vi "Twin_Simulator.vi"(6 "L2":dbl=130.0, 7 "L1":dbl=100.0, 8 "origin":cluster{"X":dbl, "Y":dbl}={"X"=200.0, "Y"=250.0}, 9 "a":dbl=20.0, 10 "beta 2":dbl(slide)=137.76536312849163 scale=-180.0..180.0, 11 "beta 1":dbl(slide)=43.24022346368716 scale=-180.0..180.0) -> (1 "3D Picture":refnum<vi>(3d-picture), 3 "Canvas":picture)   [LabVIEW 2022 SP3]
panel:
  out "A":dbl=0.009007395105217966
  out "B":dbl=1.2833295473119142
  out "L":dbl=1.2833611573405141
  out "gamma1":dbl=49.705808953024054
  out "gamma2":dbl=50.510495500567416
  out "sigma":dbl=79.87499415983615
  out "theta":dbl=0.4023432737716799
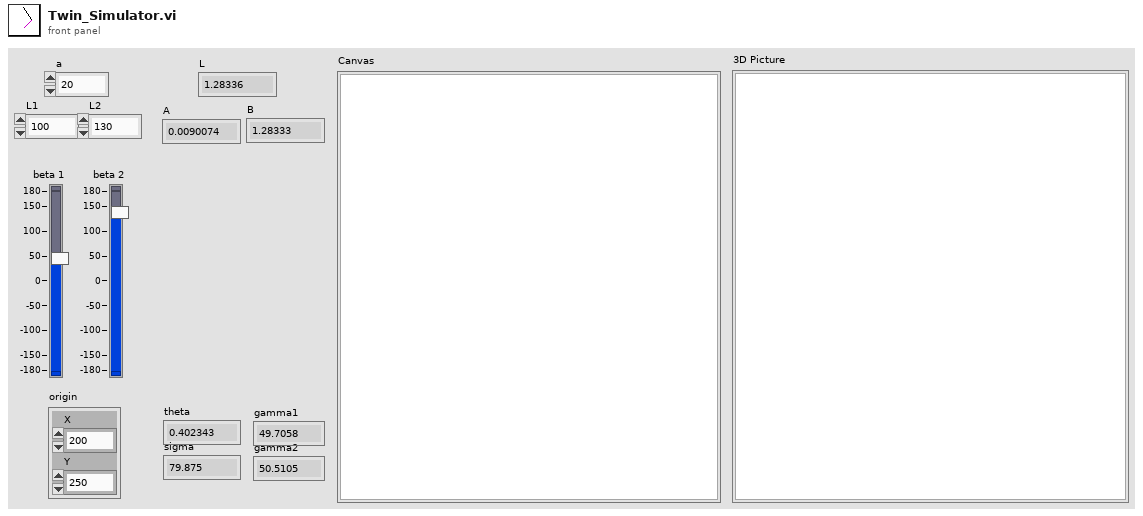
[diagram p1: front panel]
types:
  T1 = cluster{"Color":u32, "Length":dbl, "Base position":cluster{"X":dbl, "Y":dbl}, "Joint Angle":dbl}
  T2 = cluster{"Color":u32, "Length":dbl, "Base position":cluster{"X":dbl, "Y":dbl}, "Joint Angle":dbl}[]
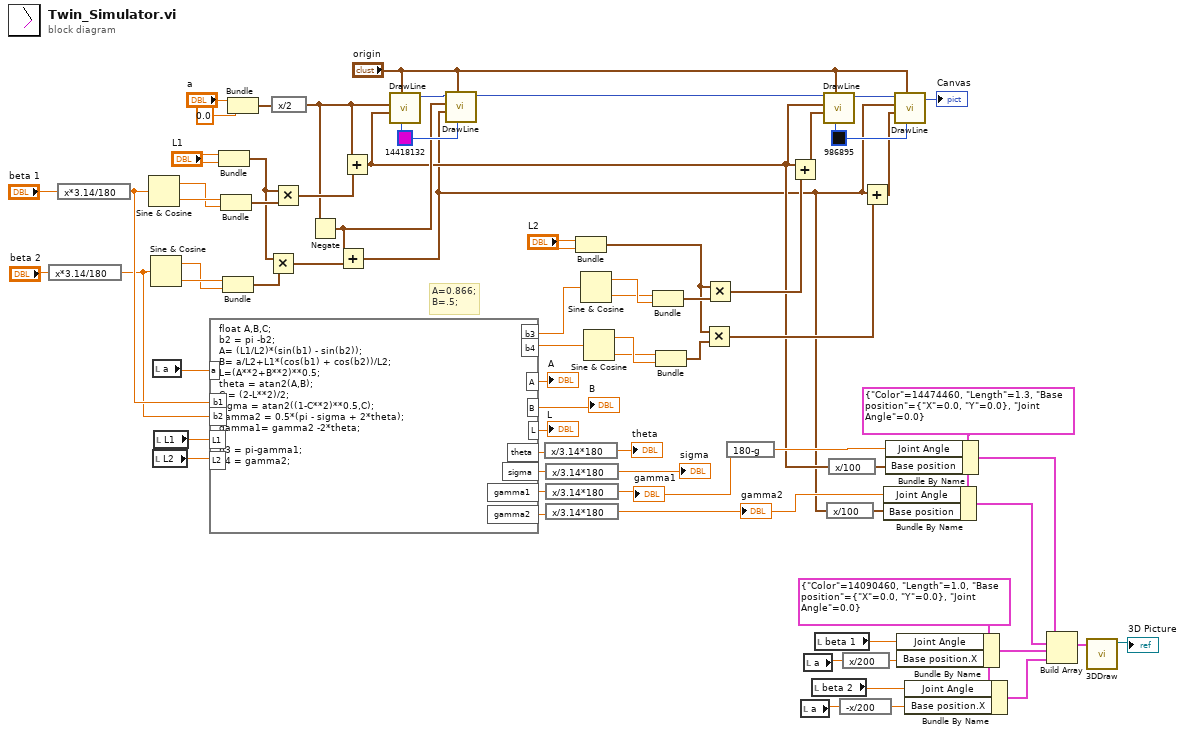
[diagram p0: block diagram]
diagram:
  w10 = T1 {"Color"=14474460, "Length"=1.3, "Base position"={"X"=0.0, "Y"=0.0}, "Joint Angle"=0.0} ("Arm")
  w14 = T1 {"Color"=14090460, "Length"=1.0, "Base position"={"X"=0.0, "Y"=0.0}, "Joint Angle"=0.0} ("Arm")
  w28 = u32 986895 ("color(black)")
  w30 = u32 14418132 ("color(black)")
  # "A=0.866;\nB=.5;"
  n1 = expression code="x*3.14/180"("beta 2") -> (w54:dbl)
  n2 = expression code="x*3.14/180"("beta 1") -> (w55:dbl)
  n3 = Sine & Cosine(0:w55) -> (1:w66:dbl, 2:w67:dbl)
  n4 = Sine & Cosine(0:w54) -> (1:w61:dbl, 2:w62:dbl)
  n5 = local read "a"() -> (w58:dbl)
  n6 = local read "L2"() -> (w56:dbl)
  n7 = local read "L1"() -> (w57:dbl)
  n8 = formula code="float A,B,C;\nb2 = pi -b2;\nA= (L1/L2)*(sin(b1) - sin(b2));\nB= a/L2+L1*(cos(b1) + cos(b2))/L2;\nL=(A**2+B**2)**0.5;\ntheta = atan2(A,B);\nC = (2-L**2)/2;\nsigma = atan2((1-C**2)**0.5,C);\ngamma2 = 0.5*(pi - sigma + 2*theta);\ngamma1= gamma2 -2*theta;\n\nb3 = pi-gamma1;\nb4 = gamma2;"("b1"=w55, "b2"=w54, "L1"=w57, "L2"=w56, "a"=w58) -> ("A"=→"A":dbl, "B"=→"B":dbl, "L"=→"L":dbl, "theta"=w53:dbl, "sigma"=w50:dbl, "gamma1"=w49:dbl, "gamma2"=w48:dbl, "b3"=w40:dbl, "b4"=w39:dbl)
  n9 = Bundle("L1"="L1", "L1"="L1") -> (w59:cluster{"L1":dbl, "L1":dbl})  [unwired: 1 in]
  n10 = Bundle(w67, w66) -> (w65:cluster{dbl, dbl})  [unwired: 1 in]
  n11 = Bundle(w62, w61) -> (w63:cluster{dbl, dbl})  [unwired: 1 in]
  n12 = Bundle("a"="a", 0.0) -> (w69:cluster{"a":dbl, dbl})  [unwired: 1 in]
  n13 = Multiply(x=w59, y=w63) -> (x*y=w37:cluster{dbl, dbl})
  n14 = expression code="x/2"(w69) -> (w32:cluster{"a":dbl, dbl})
  n15 = Multiply(x=w59, y=w65) -> (x*y=w64:cluster{dbl, dbl})
  n16 = Negate(x=w32) -> (-x=w29:cluster{"a":dbl, dbl})
  n17 = Add(x=w29, y=w37) -> (x+y=w1:cluster{dbl, dbl})
  n18 = Add(x=w32, y=w64) -> (x+y=w2:cluster{dbl, dbl})
  n19 = call "DrawLine.vi"("color(black)"=w30, "offset"="origin", "move"=w2, "start"=w32) -> ("picture out"=w31:picture)  [unwired: 7 in]
  n20 = call "DrawLine.vi"("color(black)"=w30, "offset"="origin", "move"=w1, "start"=w29, "picture in"=w31) -> ("picture out"=w26:picture)  [unwired: 6 in]
  n21 = expression code="x/3.14*180"(w53) -> (→"theta":dbl)
  n22 = expression code="x/3.14*180"(w50) -> (→"sigma":dbl)
  n23 = expression code="x/3.14*180"(w49) -> (w4:dbl)
  "gamma1" <- w4
  n24 = expression code="x/3.14*180"(w48) -> (w9:dbl)
  "gamma2" <- w9
  n25 = Bundle("L2"="L2", "L2"="L2") -> (w41:cluster{"L2":dbl, "L2":dbl})  [unwired: 1 in]
  n26 = Sine & Cosine(0:w40) -> (1:w43:dbl, 2:w42:dbl)
  n27 = Sine & Cosine(0:w39) -> (1:w47:dbl, 2:w46:dbl)
  n28 = Bundle(w42, w43) -> (w44:cluster{dbl, dbl})  [unwired: 1 in]
  n29 = Bundle(w46, w47) -> (w45:cluster{dbl, dbl})  [unwired: 1 in]
  n30 = Multiply(x=w41, y=w45) -> (x*y=w36:cluster{dbl, dbl})
  n31 = Multiply(x=w41, y=w44) -> (x*y=w38:cluster{dbl, dbl})
  n32 = expression code="180-g"(w4) -> (w3:dbl)
  n33 = Add(x=w2, y=w38) -> (x+y=w24:cluster{dbl, dbl})
  n34 = local read "a"() -> (w16:dbl)
  n35 = local read "a"() -> (w19:dbl)
  n36 = local read "beta 2"() -> (w15:dbl)
  n37 = local read "beta 1"() -> (w20:dbl)
  n38 = call "DrawLine.vi"("color(black)"=w28, "offset"="origin", "move"=w24, "start"=w2, "picture in"=w26) -> ("picture out"=w27:picture)  [unwired: 6 in]
  n39 = expression code="x/100"(w1) -> (w6:cluster{dbl, dbl})
  n40 = expression code="x/100"(w2) -> (w5:cluster{dbl, dbl})
  n41 = expression code="-x/200"(w16) -> (w17:dbl)
  n42 = expression code="x/200"(w19) -> (w18:dbl)
  n43 = Add(x=w1, y=w36) -> (x+y=w23:cluster{dbl, dbl})
  n44 = Bundle By Name(cluster=w10, "Joint Angle"=w9, "Base position"=w6) -> (w7:T1)
  n45 = Bundle By Name(cluster=w10, "Joint Angle"=w3, "Base position"=w5) -> (w8:T1)
  n46 = call "DrawLine.vi"("color(black)"=w28, "offset"="origin", "move"=w23, "start"=w1, "picture in"=w27) -> ("picture out"=→"Canvas":picture)  [unwired: 6 in]
  n47 = Bundle By Name(cluster=w14, "Joint Angle"=w20, "Base position.X"=w18) -> (w13:T1)
  n48 = Bundle By Name(cluster=w14, "Joint Angle"=w15, "Base position.X"=w17) -> (w12:T1)
  n49 = Build Array(w8, w7, w13, w12) -> (w11:T2)
  n50 = call "3DDraw.vi"("Beta/gamma"=w11) -> ("3D Picture"=→"3D Picture":refnum<vi>)  [unwired: 10 in]
